vi "RSZVB Receiver Power Calibration Harmonic.vi"(8 "error in (no error)":errorcluster {"code" format="%.0x"}, 10 "Channel (1)":i32=1, 11 "VISA session":refnum<visa-resource-name>) -> (0 "error out":errorcluster {"code" format="%.0x"}, 3 "dup VISA session":refnum<visa-resource-name>)   [LabVIEW 2011]
doc: "This VI starts the receiver calibration (2nd power calibration step for harmonic measurements), stores and applies the calibration data.\n \nNote(s):\n\n(1) For some measurements the default set timeout can be insufficient. To set higher timeout use function rszvb_setTimeOut.\n\n(2) This function is available only on R&S ZVA and ZVT instrument with K4 option installed.\n\nRemote-control command(s):\n[SENSe<Ch>:]CORRection:POWer:HARMonic:ACQuire"
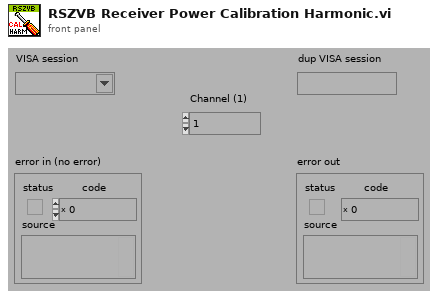
[diagram p1: front panel]
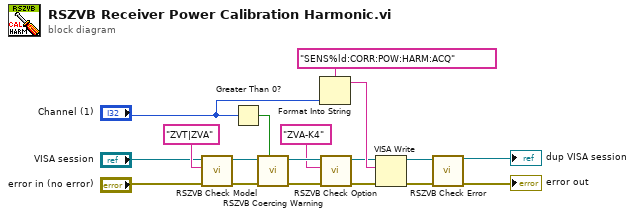
[diagram p0: block diagram]
diagram:
  n1 = call "RSZVB Check Model.vi"("error in (no error)"="error in (no error)", "Model"="ZVT|ZVA" ("Options"), "VISA session"="VISA session") -> ("error out"=w12:errorcluster, "dup VISA session"=w11:refnum<visa-resource-name>)  [unwired: 7 in]
  n2 = Greater Than 0?(x="Channel (1)") -> (x > 0?=w14:bool)
  n3 = call "RSZVB Coercing Warning.vi"("In Range?"=w14, "error in (no error)"=w12, "VISA session"=w11) -> ("error out"=w4:errorcluster, "dup VISA session"=w5:refnum<visa-resource-name>)  [unwired: 7 in]
  n4 = Format Into String(format string="SENS%ld:CORR:POW:HARM:ACQ", "Channel (1)") -> (resulting string=w15:string)  [unwired: 2 in, 1 out]
  n5 = call "RSZVB Check Option.vi"("error in (no error)"=w4, "Options"="ZVA-K4", "VISA session"=w5) -> ("error out"=w3:errorcluster, "dup VISA session"=w2:refnum<visa-resource-name>)  [unwired: 7 in]
  n6 = VISA Write(VISA resource name=w2, write buffer=w15, error in (no error)=w3) -> (VISA resource name out=w16:refnum<visa-resource-name>, error out=w17:errorcluster)  [unwired: 1 out]
  n7 = call "RSZVB Check Error.vi"("error in (no error)"=w17, "VISA session"=w16) -> ("error out"=→"error out":errorcluster, "dup VISA session"=→"dup VISA session":refnum<visa-resource-name>)  [unwired: 8 in]
